vi "XY Graph - Append Plot.vi"(8 "error in (no error)":errorcluster, 9 "Style":T1={"Plot.Anti-aliased"=FALSE, "Plot.Bar Plot Style"=0, "Plot.Digital Line Style"=0, "Plot.Digital Transition Location"=0, "Plot.Digital Transition Type"=0, "Plot.Fill To"=-1, "Plot.Fill/Point Color"=0, "Plot.Label Format"=0, "Plot.Line Style"=0, "Plot.Line Width"=0, "Plot.Plot Color"=0, "Plot.Plot Interpolation"=2, "Plot.Plot Name"="", "Plot.Point Style"=0, "Plot.Visible"=TRUE}, 10 "Data":cluster{"X":dbl[], "Y":dbl[]}, 11 "XYGraph Refnum in":refnum<vi>) -> (0 "error out":errorcluster, 3 "XYGraph Refnum out":refnum<vi>)   [LabVIEW 2016]
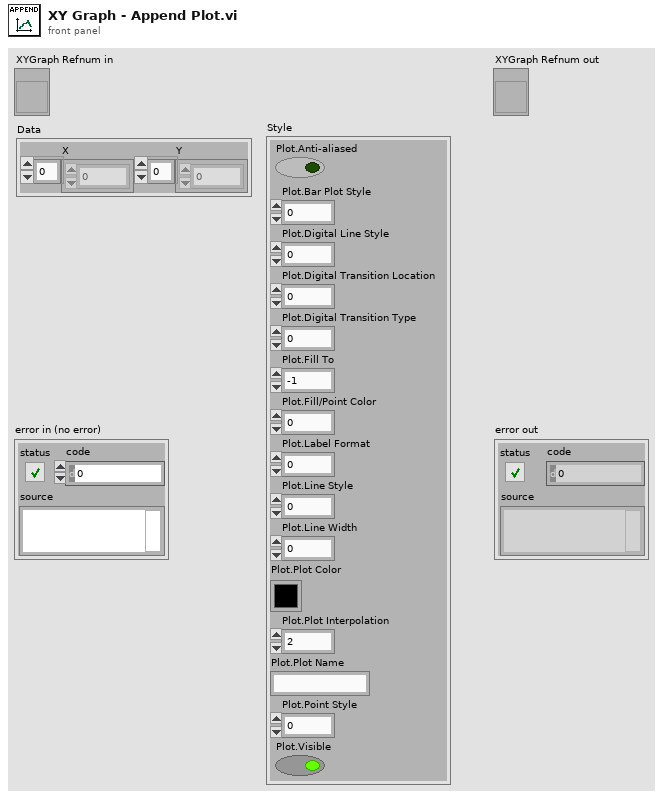
[diagram p1: front panel]
types:
  T1 = cluster{"Plot.Anti-aliased":bool, "Plot.Bar Plot Style":u8, "Plot.Digital Line Style":u8, "Plot.Digital Transition Location":u8, "Plot.Digital Transition Type":u8, "Plot.Fill To":i16, "Plot.Fill/Point Color":u32, "Plot.Label Format":u8, "Plot.Line Style":u8, "Plot.Line Width":u8, "Plot.Plot Color":u32, "Plot.Plot Interpolation":u8, "Plot.Plot Name":string, "Plot.Point Style":u8, "Plot.Visible":bool}
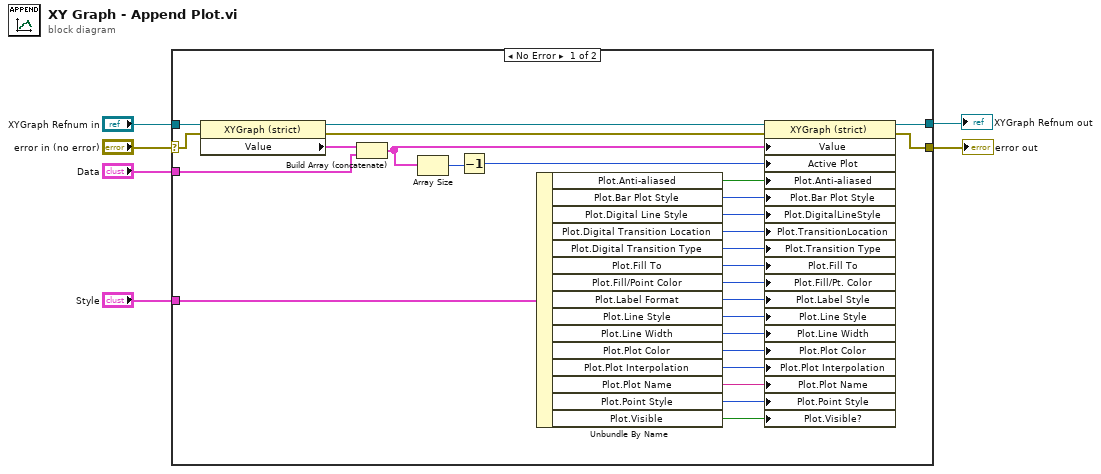
[diagram p0: block diagram]
diagram:
  n1 = case shown="No Error" "error in (no error)" {
    selector: "error in (no error)" -> [w32 w34]
    tunnel: "XYGraph Refnum in" -> [w33 w35]
    tunnel: "Data" -> [w28 _]
    tunnel: "Style" -> [w24 _]
    tunnel: [w9 w34] -> w2
    tunnel: [w8 w35] -> w1
    frame No Error {
      n2 = property class="XYGraph (strict)"(reference=w33, error in=w32) -> (reference out=w31:refnum<vi>, error out=w30:errorcluster, "Value"=w29:cluster{dbl[], dbl[]}[])
      n3 = Build Array (concatenate)(w29, w28) -> (w27:cluster{"X":dbl[], "Y":dbl[]}[])
      n4 = Array Size(array=w27) -> (size(s)=w26:i32)
      n5 = Decrement(x=w26) -> (x-1=w25:i32)
      n6 = Unbundle By Name(w24) -> ("Plot.Anti-aliased"=w23:bool, "Plot.Bar Plot Style"=w22:u8, "Plot.Digital Line Style"=w21:u8, "Plot.Digital Transition Location"=w20:u8, "Plot.Digital Transition Type"=w19:u8, "Plot.Fill To"=w18:i16, "Plot.Fill/Point Color"=w17:u32, "Plot.Label Format"=w7:u8, "Plot.Line Style"=w16:u8, "Plot.Line Width"=w15:u8, "Plot.Plot Color"=w14:u32, "Plot.Plot Interpolation"=w13:u8, "Plot.Plot Name"=w12:string, "Plot.Point Style"=w11:u8, "Plot.Visible"=w10:bool)
      n7 = property class="XYGraph (strict)"(reference=w31, error in=w30, "Value"=w27, "Active Plot"=w25, "Plot.Anti-aliased"=w23, "Plot.Bar Plot Style"=w22, "Plot.DigitalLineStyle"=w21, "Plot.TransitionLocation"=w20, "Plot.Transition Type"=w19, "Plot.Fill To"=w18, "Plot.Fill/Pt. Color"=w17, "Plot.Label Style"=w7, "Plot.Line Style"=w16, "Plot.Line Width"=w15, "Plot.Plot Color"=w14, "Plot.Plot Interpolation"=w13, "Plot.Plot Name"=w12, "Plot.Point Style"=w11, "Plot.Visible?"=w10) -> (reference out=w8:refnum<vi>, error out=w9:errorcluster)
    }
    frame Error {
    }
  }
  "XYGraph Refnum out" <- w1
  "error out" <- w2
